vi "Localization_of_Objects-1.vi"(5 "[IN] Detection Progress":refnum<vi>, 7 "[IN] Number of Frames":u32, 8 "error IN":errorcluster, 9 "[IN] Find ALL objects":bool, 10 "[IN] Movie Related Values":T2 {"Particle Fil Setups"."Type of particle filter"."Measurement Parameter" items=["Center of Mass X", "Center of Mass Y", "First Pixel X", "First Pixel Y", "Bounding Rect Left", "Bounding Rect Top", "Bounding Rect Right", "Bounding Rect Bottom", "Max Feret Diameter Start X", "Max Feret Diameter Start Y", "Max Feret Diameter End X", "Max Feret Diameter End Y", "Max Horiz. Segment Length Left", "Max Horiz. Segment Length Right", "Max Horiz. Segment Length Row", "-", "Bounding Rect Width", "Bounding Rect Height", "Bounding Rect Diagonal", "Perimeter", "Convex Hull Perimeter", "Holes' Perimeter", "Max Feret Diameter", "Equivalent Ellipse Major Axis", "Equivalent Ellipse Minor Axis", "Equivalent Ellipse Minor Axis (Feret)", "Equivalent Rect Long Side", "Equivalent Rect Short Side", "Equivalent Rect Diagonal", "Equivalent Rect Short Side (Feret)", "Average Horiz. Segment Length", "Average Vert. Segment Length", "Hydraulic Radius", "Waddel Disk Diameter", "-", "Area", "Holes' Area", "Particle & Holes' Area", "Convex Hull Area", "Image Area", "-", "Number of Holes", "Number of Horiz. Segments", "Number of Vert. Segments", "-", "Orientation", "Max Feret Diameter Orientation", "-", "% Area/Image Area", "% Area/(Particle & Holes' Area)", "Ratio of Equivalent Ellipse Axes", "Ratio of Equivalent Rect Sides", "-", "Elongation Factor", "Compactness Factor", "Heywood Circularity Factor", "Type Factor", "-", "Sum X", "Sum Y", "Sum XX", "Sum XY", "Sum YY", "Sum XXX", "Sum XXY", "Sum XYY", "Sum YYY", "-", "Moment of Inertia XX", "Moment of Inertia XY", "Moment of Inertia YY", "Moment of Inertia XXX", "Moment of Inertia XXY", "Moment of Inertia XYY", "Moment of Inertia YYY", "Norm. Moment of Inertia XX", "Norm. Moment of Inertia XY", "Norm. Moment of Inertia YY", "Norm. Moment of Inertia XXX", "Norm. Moment of Inertia XXY", "Norm. Moment of Inertia XYY", "Norm. Moment of Inertia YYY", "Hu Moment 1", "Hu Moment 2", "Hu Moment 3", "Hu Moment 4", "Hu Moment 5", "Hu Moment 6", "Hu Moment 7"]}, 11 "[IN] Localization Settings":T5 {"[IN] Image Type" items=["Grayscale (U8)", "Grayscale (I16)", "Grayscale (SGL)", "Complex (CSG)", "RGB (U32)", "HSL (U32)", "RGB (U64)", "Grayscale (U16)"]; "[IN] Particle Filter Setups"."Type of particle filter"."Measurement Parameter" items=["Center of Mass X", "Center of Mass Y", "First Pixel X", "First Pixel Y", "Bounding Rect Left", "Bounding Rect Top", "Bounding Rect Right", "Bounding Rect Bottom", "Max Feret Diameter Start X", "Max Feret Diameter Start Y", "Max Feret Diameter End X", "Max Feret Diameter End Y", "Max Horiz. Segment Length Left", "Max Horiz. Segment Length Right", "Max Horiz. Segment Length Row", "-", "Bounding Rect Width", "Bounding Rect Height", "Bounding Rect Diagonal", "Perimeter", "Convex Hull Perimeter", "Holes' Perimeter", "Max Feret Diameter", "Equivalent Ellipse Major Axis", "Equivalent Ellipse Minor Axis", "Equivalent Ellipse Minor Axis (Feret)", "Equivalent Rect Long Side", "Equivalent Rect Short Side", "Equivalent Rect Diagonal", "Equivalent Rect Short Side (Feret)", "Average Horiz. Segment Length", "Average Vert. Segment Length", "Hydraulic Radius", "Waddel Disk Diameter", "-", "Area", "Holes' Area", "Particle & Holes' Area", "Convex Hull Area", "Image Area", "-", "Number of Holes", "Number of Horiz. Segments", "Number of Vert. Segments", "-", "Orientation", "Max Feret Diameter Orientation", "-", "% Area/Image Area", "% Area/(Particle & Holes' Area)", "Ratio of Equivalent Ellipse Axes", "Ratio of Equivalent Rect Sides", "-", "Elongation Factor", "Compactness Factor", "Heywood Circularity Factor", "Type Factor", "-", "Sum X", "Sum Y", "Sum XX", "Sum XY", "Sum YY", "Sum XXX", "Sum XXY", "Sum XYY", "Sum YYY", "-", "Moment of Inertia XX", "Moment of Inertia XY", "Moment of Inertia YY", "Moment of Inertia XXX", "Moment of Inertia XXY", "Moment of Inertia XYY", "Moment of Inertia YYY", "Norm. Moment of Inertia XX", "Norm. Moment of Inertia XY", "Norm. Moment of Inertia YY", "Norm. Moment of Inertia XXX", "Norm. Moment of Inertia XXY", "Norm. Moment of Inertia XYY", "Norm. Moment of Inertia YYY", "Hu Moment 1", "Hu Moment 2", "Hu Moment 3", "Hu Moment 4", "Hu Moment 5", "Hu Moment 6", "Hu Moment 7"]}) -> (0 "error OUT":errorcluster, 2 "[OUT] Movie Related Values":T2 {"Particle Fil Setups"."Type of particle filter"."Measurement Parameter" items=["Center of Mass X", "Center of Mass Y", "First Pixel X", "First Pixel Y", "Bounding Rect Left", "Bounding Rect Top", "Bounding Rect Right", "Bounding Rect Bottom", "Max Feret Diameter Start X", "Max Feret Diameter Start Y", "Max Feret Diameter End X", "Max Feret Diameter End Y", "Max Horiz. Segment Length Left", "Max Horiz. Segment Length Right", "Max Horiz. Segment Length Row", "-", "Bounding Rect Width", "Bounding Rect Height", "Bounding Rect Diagonal", "Perimeter", "Convex Hull Perimeter", "Holes' Perimeter", "Max Feret Diameter", "Equivalent Ellipse Major Axis", "Equivalent Ellipse Minor Axis", "Equivalent Ellipse Minor Axis (Feret)", "Equivalent Rect Long Side", "Equivalent Rect Short Side", "Equivalent Rect Diagonal", "Equivalent Rect Short Side (Feret)", "Average Horiz. Segment Length", "Average Vert. Segment Length", "Hydraulic Radius", "Waddel Disk Diameter", "-", "Area", "Holes' Area", "Particle & Holes' Area", "Convex Hull Area", "Image Area", "-", "Number of Holes", "Number of Horiz. Segments", "Number of Vert. Segments", "-", "Orientation", "Max Feret Diameter Orientation", "-", "% Area/Image Area", "% Area/(Particle & Holes' Area)", "Ratio of Equivalent Ellipse Axes", "Ratio of Equivalent Rect Sides", "-", "Elongation Factor", "Compactness Factor", "Heywood Circularity Factor", "Type Factor", "-", "Sum X", "Sum Y", "Sum XX", "Sum XY", "Sum YY", "Sum XXX", "Sum XXY", "Sum XYY", "Sum YYY", "-", "Moment of Inertia XX", "Moment of Inertia XY", "Moment of Inertia YY", "Moment of Inertia XXX", "Moment of Inertia XXY", "Moment of Inertia XYY", "Moment of Inertia YYY", "Norm. Moment of Inertia XX", "Norm. Moment of Inertia XY", "Norm. Moment of Inertia YY", "Norm. Moment of Inertia XXX", "Norm. Moment of Inertia XXY", "Norm. Moment of Inertia XYY", "Norm. Moment of Inertia YYY", "Hu Moment 1", "Hu Moment 2", "Hu Moment 3", "Hu Moment 4", "Hu Moment 5", "Hu Moment 6", "Hu Moment 7"]})   [LabVIEW 2017]
doc: "This \"header\" subVI merges the subprograms for localization of objects and saving of their properties (areas, centers of masses)"
uses:
  <vilib>/vision/Avi.llb/IMAQ AVI2 Refnum.ctl
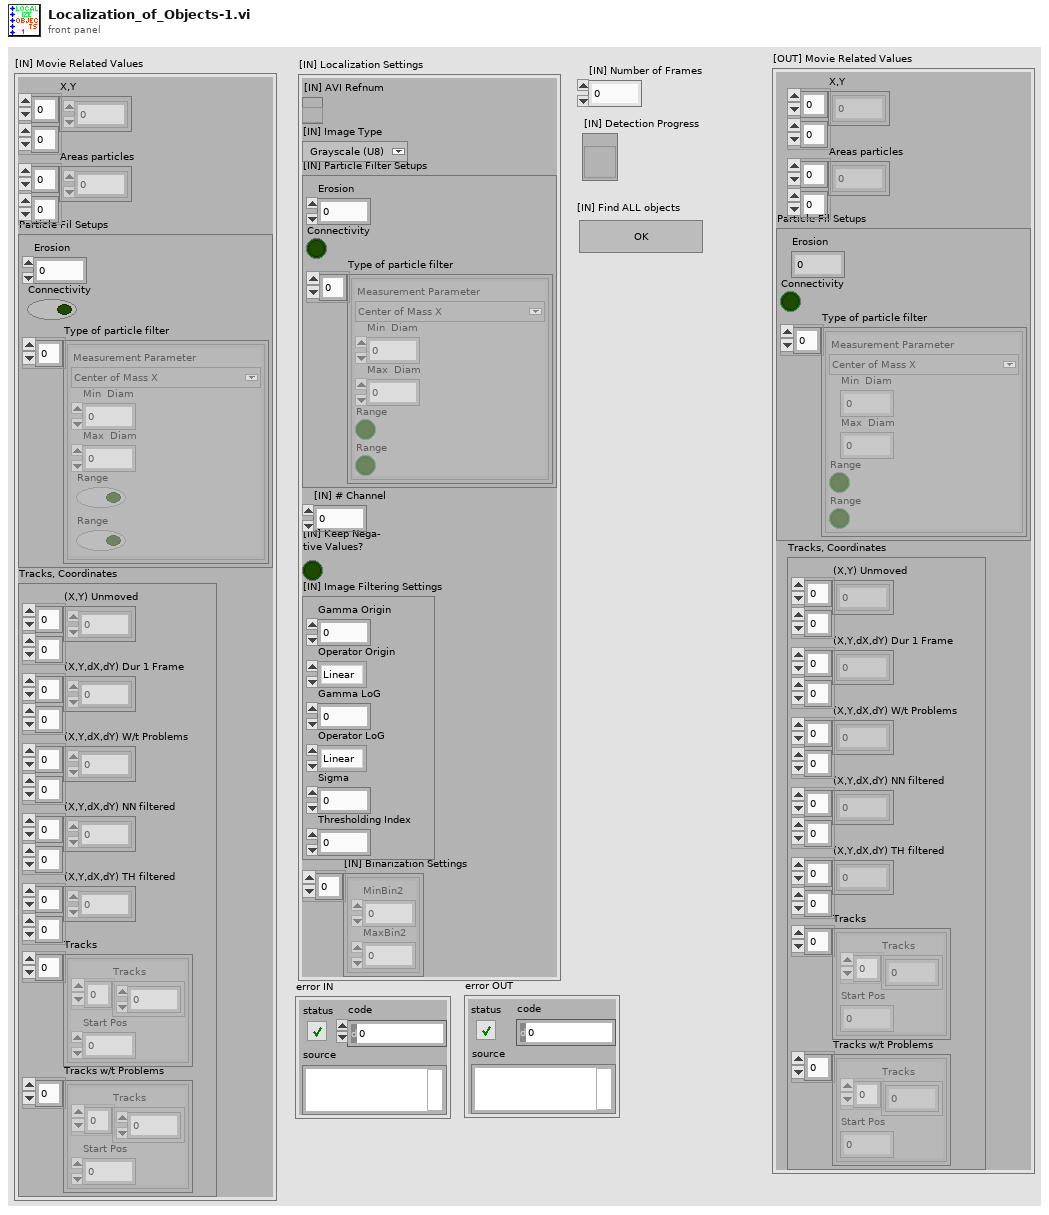
[diagram p1: front panel]
types:
  T1 = typedef "Particle Parameters" = i32
  T2 = cluster{"X,Y":dbl[][], "Areas particles":dbl[][], "Particle Fil Setups":cluster{"Erosion":i32, "Connectivity ":bool, "Type of particle filter":cluster{"Measurement Parameter":T1, "Min  Diam":dbl, "Max  Diam":dbl, "Range":bool, "Range":bool}[]}, "Tracks, Coordinates":cluster{"(X,Y) Unmoved":dbl[][], "(X,Y,dX,dY) Dur 1 Frame":dbl[][], "(X,Y,dX,dY) W/t Problems":dbl[][], "(X,Y,dX,dY) NN filtered":dbl[][], "(X,Y,dX,dY) TH filtered":dbl[][], "Tracks":cluster{"Tracks":dbl[], "Start Pos":i32}[], "Tracks w/t Problems":cluster{"Tracks":dbl[], "Start Pos":i32}[]}}
  T3 = typedef "IMAQ AVI2 Refnum.ctl" = refnum<k20>
  T4 = typedef "Image Type" = u32
  T5 = cluster{"[IN] AVI Refnum":T3, "[IN] Image Type":T4, "[IN] Particle Filter Setups":cluster{"Erosion":i32, "Connectivity ":bool, "Type of particle filter":cluster{"Measurement Parameter":T1, "Min  Diam":dbl, "Max  Diam":dbl, "Range":bool, "Range":bool}[]}, "[IN] # Channel":u8, "[IN] Keep Nega-\ntive Values?":bool, "[IN] Image Filtering Settings":cluster{"Gamma Origin":sgl, "Operator Origin":enum32{"Linear", "Log", "Exp", "Square", "Square root", "Power X", "Power 1/X"}, "Gamma LoG":sgl, "Operator LoG":enum32{"Linear", "Log", "Exp", "Square", "Square root", "Power X", "Power 1/X"}, "Sigma":dbl, "Thresholding Index":i8}, "[IN] Binarization Settings":cluster{"MinBin2":sgl, "MaxBin2":sgl}[]}
  T6 = cluster{"Erosion":i32, "Connectivity ":bool, "Type of particle filter":cluster{"Measurement Parameter":T1, "Min  Diam":dbl, "Max  Diam":dbl, "Range":bool, "Range":bool}[]}
  T7 = cluster{"Gamma Origin":sgl, "Operator Origin":enum32{"Linear", "Log", "Exp", "Square", "Square root", "Power X", "Power 1/X"}, "Gamma LoG":sgl, "Operator LoG":enum32{"Linear", "Log", "Exp", "Square", "Square root", "Power X", "Power 1/X"}, "Sigma":dbl, "Thresholding Index":i8}
  T8 = cluster{"Points (X,Y)":dbl[], "Areas of points (X,Y)":dbl[]}[]
  T9 = typedef "IMAQ Image.ctl" = refnum<image>
  T10 = cluster{"Points (X,Y)":dbl[], "Areas of points (X,Y)":dbl[]}
  T11 = cluster{"Area":dbl, "Number of Holes":dbl, "Bounding Rect":cluster{"Left":dbl, "Top":dbl, "Right":dbl, "Bottom":dbl}, "Center of Mass":cluster{"X":dbl, "Y":dbl}, "Orientation":dbl, "Dimensions":cluster{"Width":dbl, "Height":dbl}}[]
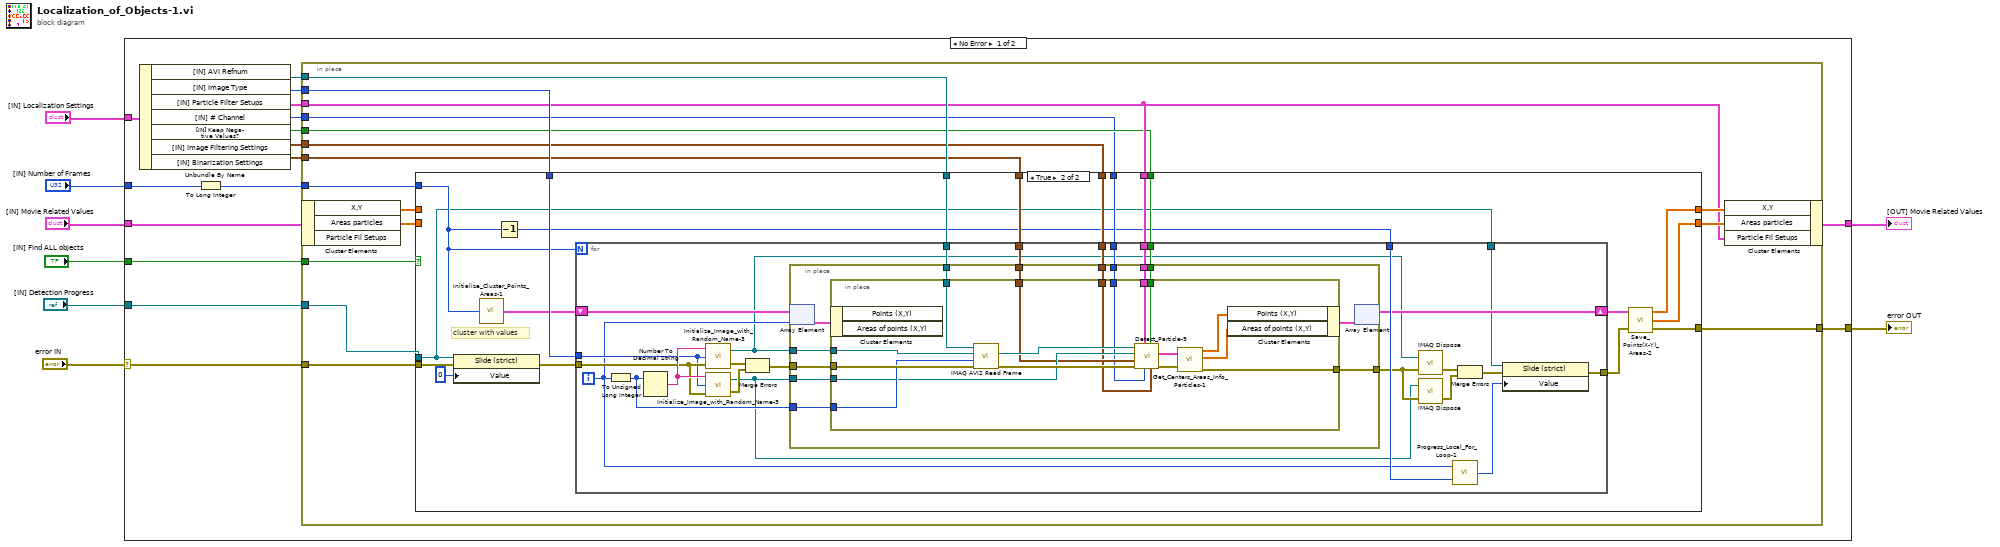
[diagram p0: block diagram]
diagram:
  n1 = case shown="No Error" "error IN" {
    selector: "error IN" -> [w14 w120]
    tunnel: "[IN] Movie Related Values" -> [w24 w119]
    tunnel: "[IN] Find ALL objects" -> [w23 _]
    tunnel: "[IN] Localization Settings" -> [w22 _]
    tunnel: "[IN] Number of Frames" -> [w12 _]
    tunnel: "[IN] Detection Progress" -> [w11 _]
    tunnel: [w10 w120] -> w2
    tunnel: [w9 w119] -> w1
    frame No Error {
      n2 = Unbundle By Name(w22) -> ("[IN] AVI Refnum"=w21:T3, "[IN] Image Type"=w20:T4, "[IN] Particle Filter Setups"=w19:T6, "[IN] # Channel"=w18:u8, "[IN] Keep Nega-\ntive Values?"=w17:bool, "[IN] Image Filtering Settings"=w16:T7, "[IN] Binarization Settings"=w15:cluster{"MinBin2":sgl, "MaxBin2":sgl}[])
      n3 = To Long Integer(number=w12) -> (32bit integer=w13:i32)
      n4 = in-place {
        in-place-border: w23 -> [w40]
        in-place-border: w21 -> [w31]
        in-place-border: w20 -> [w32]
        in-place-border: w19 -> [w29]
        in-place-border: w18 -> [w27]
        in-place-border: w17 -> [w28]
        in-place-border: w16 -> [w26]
        in-place-border: w15 -> [w30]
        in-place-border: w13 -> [w35]
        in-place-border: w14 -> [w34]
        in-place-border: w11 -> [w33]
        in-place-border: [w25] -> w10
        n5 = in-place-cluster #1(w24) -> ("X,Y"=w39:dbl[][], "Areas particles"=w38:dbl[][])  [unwired: 1 out]
        n6 = case shown="True" w40 {
          tunnel: w39 -> [w43 _]
          tunnel: w38 -> [w42 _]
          tunnel: [w43 w46] -> w37
          tunnel: [w42 w45] -> w36
          tunnel: w35 -> [_ w51]
          tunnel: w34 -> [w41 w62]
          tunnel: w33 -> [_ w49]
          tunnel: w32 -> [_ w59]
          tunnel: w31 -> [_ w57]
          tunnel: w30 -> [_ w56]
          tunnel: w29 -> [_ w55]
          tunnel: w28 -> [_ w54]
          tunnel: w27 -> [_ w53]
          tunnel: w26 -> [_ w52]
          tunnel: [w41 w44] -> w25
          frame False {
          }
          frame True {
            # "cluster with values"
            n7 = property on="Property Node" class="Slide (strict)"(reference=w49, error in=w62, "Value"=u8 0) -> (error out=w60:errorcluster)  [unwired: 1 out]
            n8 = call "Initialize_Cluster_Points_Areas-1.vi"("[IN] Number of frames"=w51) -> ("[OUT] Cluster of \npoints and areas"=w58:T8)
            n9 = Decrement(x=w51) -> (x-1=w50:i32)
            n10 = for {
              N: w51 -> [_]
              tunnel: w60 -> [w87]
              tunnel: w59 -> [w86]
              shift-right: [w70] -> w48
              shift-left: w58 -> [w81]
              tunnel: w57 -> [w78]
              tunnel: w56 -> [w77]
              tunnel: w55 -> [w76]
              tunnel: w54 -> [w75]
              tunnel: w53 -> [w74]
              tunnel: w52 -> [w73]
              tunnel: w50 -> [w72]
              tunnel: w49 -> [w64]
              tunnel: [w63] -> w47
              i -> [w71]
              n11 = To Unsigned Long Integer(number=w71) -> (unsigned 32bit integer=w79:u32)
              n12 = Number To Decimal String(number=w79) -> (decimal integer string=w88:string)  [unwired: 1 in]
              n13 = call "Initialize_Image_with_Random_Name-3.vi"("error IN"=w87, "Image Type"=w86, "Unique ID"=w88) -> ("error OUT"=w85:errorcluster, "[OUT] New Image"=w67:T9)
              n14 = call "Initialize_Image_with_Random_Name-3.vi"("error IN"=w87, "Image Type"=w86, "Unique ID"=w88) -> ("error OUT"=w84:errorcluster, "[OUT] New Image"=w68:T9)
              n15 = Merge Errors(w85, w84) -> (w80:errorcluster)
              n16 = in-place {
                in-place-border: w80 -> [w100]
                in-place-border: w67 -> [w98]
                in-place-border: w68 -> [w97]
                in-place-border: w79 -> [w96]
                in-place-border: w78 -> [w95]
                in-place-border: w77 -> [w94]
                in-place-border: w76 -> [w93]
                in-place-border: w75 -> [w92]
                in-place-border: w74 -> [w91]
                in-place-border: w73 -> [w90]
                in-place-border: [w89] -> w69
                n17 = in-place-array #2(w81, w71) -> (w101:T10)
                n18 = in-place {
                  in-place-border: w100 -> [w118]
                  in-place-border: w98 -> [w116]
                  in-place-border: w97 -> [w112]
                  in-place-border: w96 -> [w117]
                  in-place-border: w95 -> [w115]
                  in-place-border: w94 -> [w111]
                  in-place-border: w93 -> [w110]
                  in-place-border: w92 -> [w109]
                  in-place-border: w91 -> [w108]
                  in-place-border: w90 -> [w107]
                  in-place-border: [w102] -> w89
                  n19 = in-place-cluster #3(w101) -> ()  [unwired: 2 out]
                  n20 = call "IMAQ AVI2 Read Frame"("error in (no error)"=w118, "Frame Number"=w117, "Image"=w116, "AVI Refnum"=w115) -> ("error out"=w114:errorcluster, "Image Out"=w113:T9)  [unwired: 5 in, 1 out]
                  n21 = call "Detect_Particle-9.vi"("[IN] Image Filtering Settings"=w107, "Keep Nega-\ntive Values?"=w109, "# Channel"=w108, "Particle Searching Settings"=w110, "error IN"=w114, "[IN] Binarization Settings"=w111, "[IN] Destination Image"=w112, "[IN] Frame"=w113) -> ("error OUT"=w105:errorcluster, "[OUT] Particle Reports (Pixels)"=w106:T11)  [unwired: 1 in, 1 out]
                  n22 = call "Get_Centers_Areas_Info_Particles-1.vi"("[IN] Particle Reports (Pixels)"=w106, "error in"=w105) -> ("[OUT] Array of X,Y"=w104:dbl[], "[OUT] Array of Area"=w103:dbl[], "error out"=w102:errorcluster)  [unwired: 1 out]
                  n23 = in-place-cluster #3("Points (X,Y)"=w104, "Areas of points (X,Y)"=w103) -> (w99:T10)
                }
                n24 = in-place-array #2(w99) -> (w70:T8)  [unwired: 1 out]
              }
              n25 = call "IMAQ Dispose"("Image"=w67, "error in (no error)"=w69) -> ("error out"=w83:errorcluster)  [unwired: 4 in]
              n26 = call "IMAQ Dispose"("Image"=w68, "error in (no error)"=w69) -> ("error out"=w82:errorcluster)  [unwired: 4 in]
              n27 = call "Progress_Local_For_Loop-1.vi"("[IN] Number of Frames"=w72, "[IN] Current Index"=w71) -> ("[OUT] % progress"=w65:u8)
              n28 = Merge Errors(w83, w82) -> (w66:errorcluster)
              n29 = property on="Property Node" class="Slide (strict)"(reference=w64, error in=w66, "Value"=w65) -> (error out=w63:errorcluster)  [unwired: 1 out]
            }
            n30 = call "Save_Points(X-Y)_Areas-2.vi"("error IN"=w47, "[IN] Cluster of \npoints and areas"=w48) -> ("error OUT"=w44:errorcluster, "[OUT] Areas"=w45:dbl[][], "[OUT] Points (X,Y)"=w46:dbl[][])  [unwired: 1 in]
          }
        }
        n31 = in-place-cluster #1("X,Y"=w37, "Areas particles"=w36, "Particle Fil Setups"=w29) -> (w9:T2)
      }
    }
    frame Error {
    }
  }
  "error OUT" <- w2
  "[OUT] Movie Related Values" <- w1
